vi "8164B Whait till Done.vi"(8 "error in":errorcluster, 9 "timeout ms":i32=1000, 11 "KeySight 8164B control in":T1) -> (0 "error out":errorcluster, 3 "KeySight 8164B control out":T1)   [LabVIEW 2018, in "KeySight 8164B LAN InstrLib.lvlib"]
uses:
  KeySight 8164B LAN InstrLib.lvlib
  typedefs/KeySight 8164B control.ctl
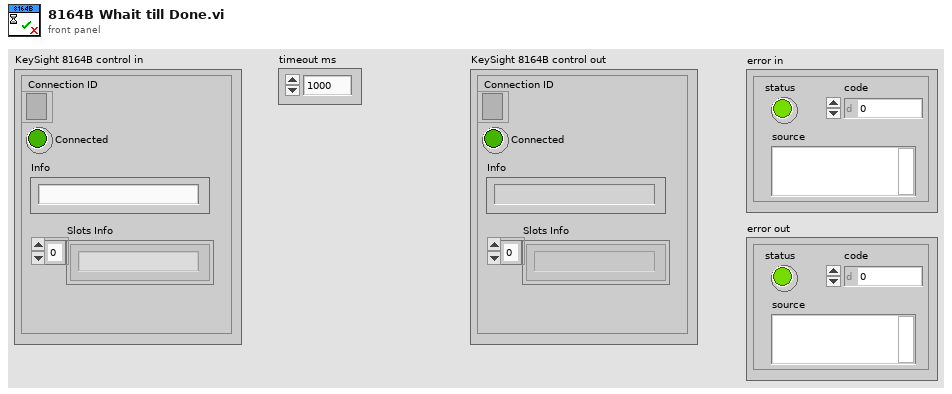
[diagram p1: front panel]
types:
  T1 = typedef "KeySight 8164B LAN InstrLib.lvlib/KeySight 8164B control.ctl" = cluster{"Connection ID":refnum<k5>, "Connected":bool, "Info":string, "Slots Info":string[]}
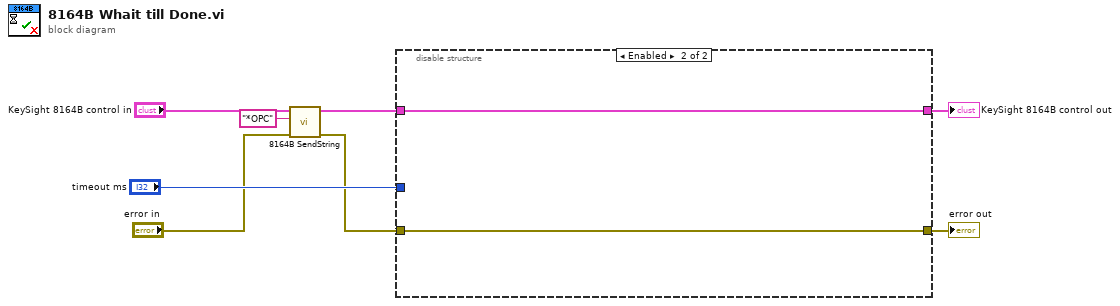
[diagram p0: block diagram]
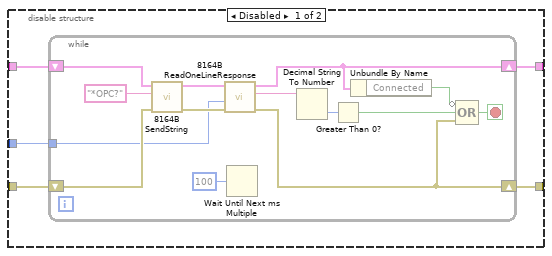
[diagram p2: hidden frame]
diagram:
  n1 = call "8164B SendString.vi"("error in"="error in", "CMD"="*OPC", "KeySight 8164B control in"="KeySight 8164B control in") -> ("error out"=w2:errorcluster, "KeySight 8164B control out"=w4:T1)  [unwired: 7 in]
  n2 = disable-structure shown="Enabled" {
    disable-tunnel: [w13 w28] -> w8
    disable-tunnel: [w12 w29] -> w7
    disable-tunnel: "timeout ms" -> [w11 _]
    disable-tunnel: w4 -> [w10 w29]
    disable-tunnel: w2 -> [w9 w28]
    frame Disabled {
      n3 = while {
        shift-right: [w15] -> w12
        shift-left: w10 -> [w27]
        shift-right: [w17] -> w13
        shift-left: w9 -> [w26]
        tunnel: w11 -> [w16]
        stop <- w18 stop-if-true
        n4 = call "8164B SendString.vi"("error in"=w26, "CMD"="*OPC?", "KeySight 8164B control in"=w27) -> ("error out"=w23:errorcluster, "KeySight 8164B control out"=w24:T1)  [unwired: 7 in]
        n5 = call "8164B ReadOneLineResponse.vi"("error in"=w23, "timeout ms"=w16, "KeySight 8164B control in"=w24) -> ("error out"=w17:errorcluster, "OneLineResponse"=w22:string, "KeySight 8164B control out"=w15:T1)  [unwired: 6 in]
        n6 = Wait Until Next ms Multiple(millisecond multiple=u32 100) -> ()  [unwired: 1 out]
        n7 = Decimal String To Number(string=w22) -> (number=w21:i32)  [unwired: 2 in, 1 out]
        n8 = Greater Than 0?(x=w21) -> (x > 0?=w20:bool)
        n9 = Unbundle By Name(w15) -> ("Connected"=w14:bool)
        n10 = Compound Arithmetic op=OR(invert w14, w20, w17) -> (w18:bool)
      }
    }
    frame Enabled {
    }
  }
  "KeySight 8164B control out" <- w7
  "error out" <- w8
